vi "LoadLiftMotorValues.vi"(8 "error in":errorcluster) -> (0 "error out":errorcluster)   [LabVIEW 2015]
uses:
  Drive/Implementation/Advanced Drive VIs/PID Type Def.ctl
  <vilib>/Rock Robotics/Network Tables/NT Read Numeric Array.vi
  Lift/TW Global.vi
panel:
  out "Settings":cluster{"Tape Increments (in)":dbl}
  out "PID":T1
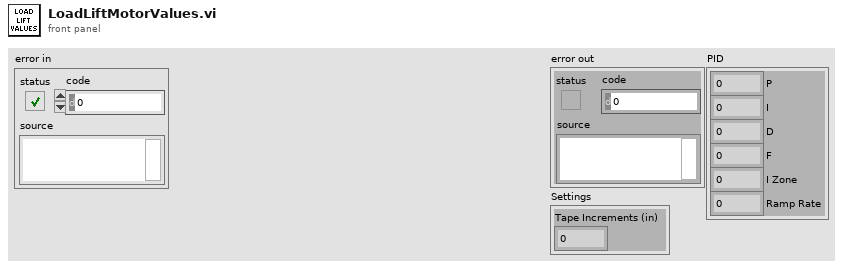
[diagram p1: front panel]
types:
  T1 = typedef "PID Type Def.ctl" = cluster{"P":dbl, "I":dbl, "D":dbl, "F":dbl, "I Zone":dbl, "Ramp Rate":dbl}
  T2 = typedef "Detailed Motor Type Def.ctl" = cluster{"MotorRef":T3, "Encoder Ticks Per Rev":dbl, "Set Position":dbl, "Wheel Radius":dbl}
  T3 = typedef "WPI_MotorControlDeviceRef.ctl" = cluster{"DeviceStatus":errorcluster, "Type":T4, "PWM":cluster{"PWM Channel":T5, "DeadBand":T6}, "CAN":cluster{"Device Number":u8, "Control Mode":T7, "Semaphore":T8, "Max Vout":dbl, "TalonSRX Control Mode":T9}, "Invert":bool}
  T4 = typedef "WPI_MotorControlType.ctl" = enum16{"PWM", "CAN", "CANTalonSRX"}
  T5 = typedef "FPGA_DIOPWMChannel.ctl" = enum8{"PWM 0", "PWM 1", "PWM 2", "PWM 3", "PWM 4", "PWM 5", "PWM 6", "PWM 7", "PWM 8", "PWM 9", "PWM MXP 0", "PWM MXP 1", "PWM MXP 2", "PWM MXP 3", "PWM MXP 4", "PWM MXP 5", "PWM MXP 6", "PWM MXP 7", "PWM MXP 8", "PWM MXP 9", "Invalid"}
  T6 = typedef "WPI_PWMDeadband.ctl" = cluster{"Name":string, "maxPositivePwm":i32, "minPositivePwm":i32, "centerPwm":i32, "maxNegativePwm":i32, "minNegativePwm":i32, "angularRange":u16}
  T7 = typedef "WPI_CANJaguar_ControlMode.ctl" = enum8{"Percent VBus", "Current", "Speed", "Position", "Voltage"}
  T8 = typedef "Semaphore RefNum" = refnum<k1>
  T9 = typedef "WPI_CANTalonSRX_APIControlMode.ctl" = enum8{"Percent VBus", "Speed", "Position", "Slave", "Unchanged / Invalid", "Voltage Compensation", "Current", "Motion Profile"}
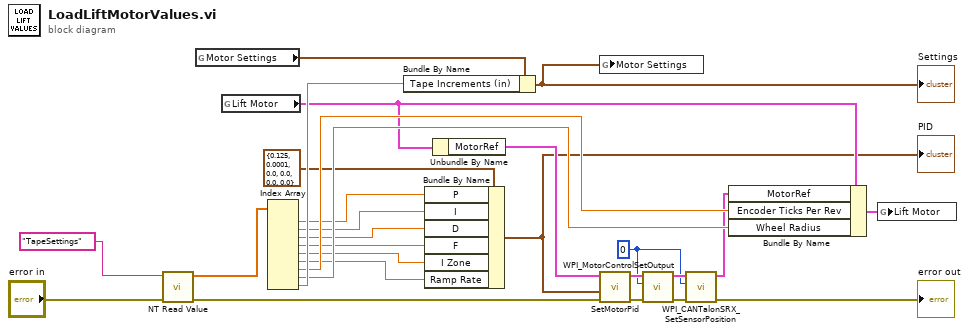
[diagram p0: block diagram]
diagram:
  w4 = 0
  n1 = call-poly <vilib>:"NT Read Value.vi"("error in"="error in", "Name"="TapeSettings") -> ("error out"=w8:errorcluster, "Numeric Array"=w11:dbl[])  [unwired: 8 in]
  n2 = global read "TW Global.vi" "Motor Settings"() -> (w26:cluster{"Tape Increments (in)":dbl})
  n3 = global read "TW Global.vi" "Lift Motor"() -> (w21:T2)
  n4 = Index Array(array=w11) -> (element #1=w13:dbl, element #2=w14:dbl, element #3=w15:dbl, element #4=w16:dbl, element #5=w17:dbl, element #6=w18:dbl, element #7=w22:dbl, element #8=w23:dbl, element #9=w27:dbl)  [unwired: 9 in]
  n5 = Bundle By Name(cluster=w26, "Tape Increments (in)"=w27) -> (w25:cluster{"Tape Increments (in)":dbl})
  "Settings" <- w25
  n6 = Bundle By Name(cluster=T1 {"P"=0.125, "I"=0.0001, "D"=0.0, "F"=0.0, "I Zone"=0.0, "Ramp Rate"=0.0} ("PID"), "P"=w13, "I"=w14, "D"=w15, "F"=w16, "I Zone"=w17, "Ramp Rate"=w18) -> (w19:T1)
  "PID" <- w19
  n7 = Unbundle By Name(w21) -> ("MotorRef"=w20:T3)
  n8 = global write "TW Global.vi" "Motor Settings"(w25) -> ()
  n9 = call "SetMotorPid.vi"("error in (no error)"=w8, "PID"=w19, "Motor Ref In"=w20) -> ("error out"=w3:errorcluster, "Motor Ref Out"=w5:T3)  [unwired: 7 in]
  n10 = call <vilib>:"WPI_MotorControlSetOutput.vi"("error in (no error)"=w3, "Output"=w4, "MotorControlDevRef"=w5) -> ("error out"=w2:errorcluster, "MotorControlDevRef"=w7:T3)  [unwired: 6 in, 1 out]
  n11 = call <vilib>:"WPI_CANTalonSRX_SetSensorPosition.vi"("error in (no error)"=w2, "New Sensor Position"=w4, "CAN Talon SRX Ref"=w7) -> ("error out"=→"error out":errorcluster, "CAN Talon SRX Ref"=w6:T3)  [unwired: 7 in]
  n12 = Bundle By Name(cluster=w21, "MotorRef"=w6, "Encoder Ticks Per Rev"=w22, "Wheel Radius"=w23) -> (w24:T2)
  n13 = global write "TW Global.vi" "Lift Motor"(w24) -> ()
